vi "ex7.vi"() -> ()   [LabVIEW 2020]
uses:
  <vilib>/measure/madcrms.llb/Basic Averaged DC-RMS for N Chan.vi
  <vilib>/measure/NI_MAPro.lvlib
panel:
  out "greater than 3":bool
  out "amlitude":dbl
  out "frequency":dbl
  out "ofset":dbl
  out "Waveform Graph":dynamicdata(graph)
  in  "samples":dbl
  in  "Fs":dbl
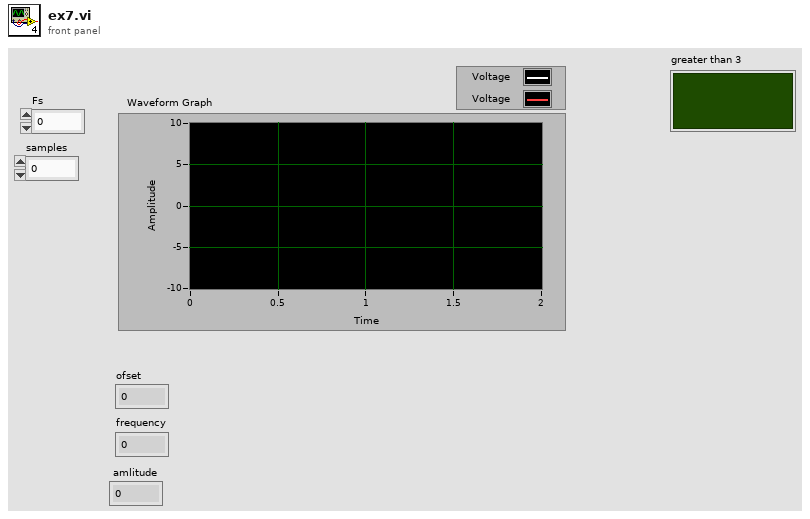
[diagram p1: front panel]
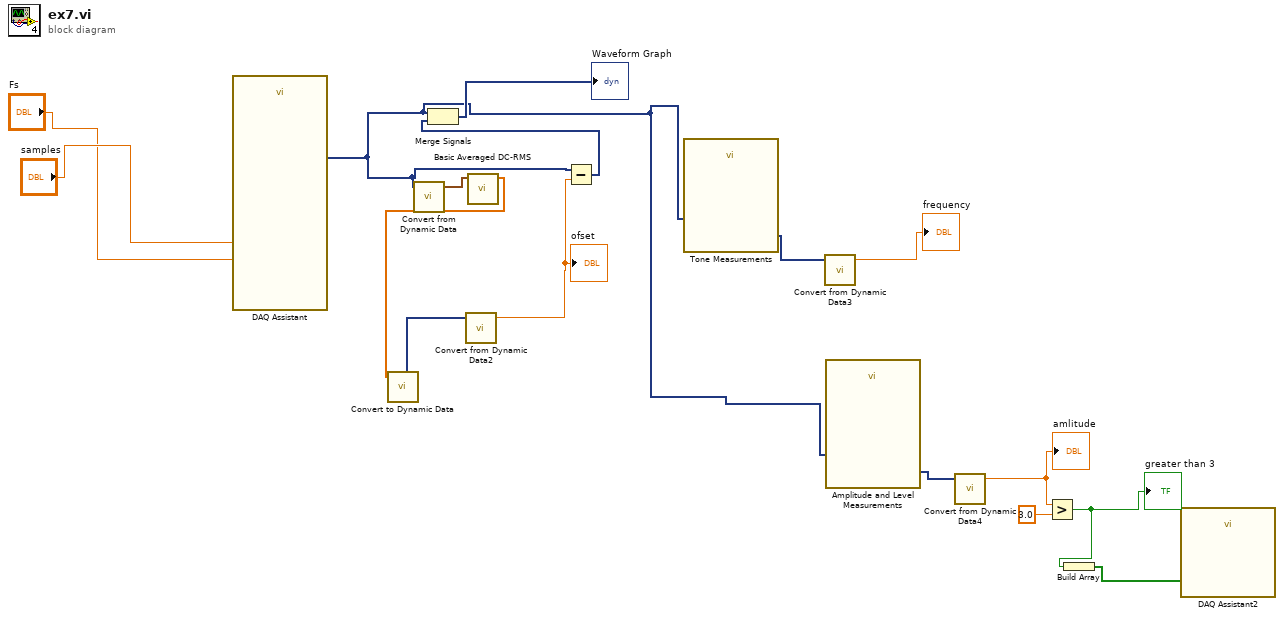
[diagram p0: block diagram]
diagram:
  n1 = call "DAQ Assistant"("rate"="Fs", "number of samples"="samples") -> ("data"=w3:dynamicdata)  [unwired: 15 in, 2 out]
  n2 = call "Convert from Dynamic Data"("Dynamic Data Type"=w3) -> ("Array of Waveform"=w15:waveform(dbl)[])  [unwired: 3 in]
  n3 = call-poly <vilib>:"Basic Averaged DC-RMS.vi"("signals in"=w15) -> ("DC values"=w1:dbl[])  [unwired: 7 in, 3 out]
  n4 = call "Convert to Dynamic Data"("Array"=w1) -> ("Dynamic Data Type"=w14:dynamicdata)  [unwired: 3 in]
  n5 = call "Convert from Dynamic Data2"("Dynamic Data Type"=w14) -> ("Scalar"=w13:dbl)  [unwired: 3 in]
  "ofset" <- w13
  n6 = Subtract(x=w3, y=w13) -> (x-y=w4:dynamicdata)
  n7 = Merge Signals(w3, w4) -> (→"Waveform Graph":dynamicdata)
  n8 = call "Tone Measurements"("Signals"=w3) -> ("Frequency"=w11:dynamicdata)  [unwired: 9 in, 1 out]
  n9 = call "Convert from Dynamic Data3"("Dynamic Data Type"=w11) -> ("Scalar"=→"frequency":dbl)  [unwired: 3 in]
  n10 = call "Amplitude and Level Measurements"("Signals"=w3) -> ("RMS"=w2:dynamicdata)  [unwired: 13 in, 1 out]
  n11 = call "Convert from Dynamic Data4"("Dynamic Data Type"=w2) -> ("Scalar"=w8:dbl)  [unwired: 3 in]
  "amlitude" <- w8
  n12 = Greater?(x=w8, y=3.0) -> (0:w5:bool)
  "greater than 3" <- w5
  n13 = Build Array(w5) -> (w6:bool[])
  n14 = call "DAQ Assistant2"("data"=w6) -> ()  [unwired: 17 in, 2 out]
